vi "2015 Dumping.vi"(6 "Scoop angle":dbl format="%#_13g", 7 "Drum angle":dbl format="%#_13g", 8 "Winch angle":dbl, 9 "Dump":bool) -> (0 "Dumping Completed":bool, 1 "Drum PW":dbl format="%#_13g", 2 "Winch PW":dbl format="%#_13g", 3 "Scoop PW":dbl format="%#_13g")   [LabVIEW 2014]
panel:
  out "Numeric 2":i32
  out "Numeric":i32
  out "Boolean":bool
  out "Dump behav":bool
  out "D, S, W Aligned":bool
  # "Test indicators"
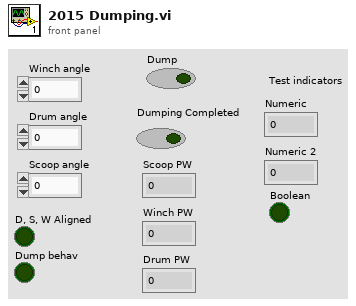
[diagram p1: front panel]
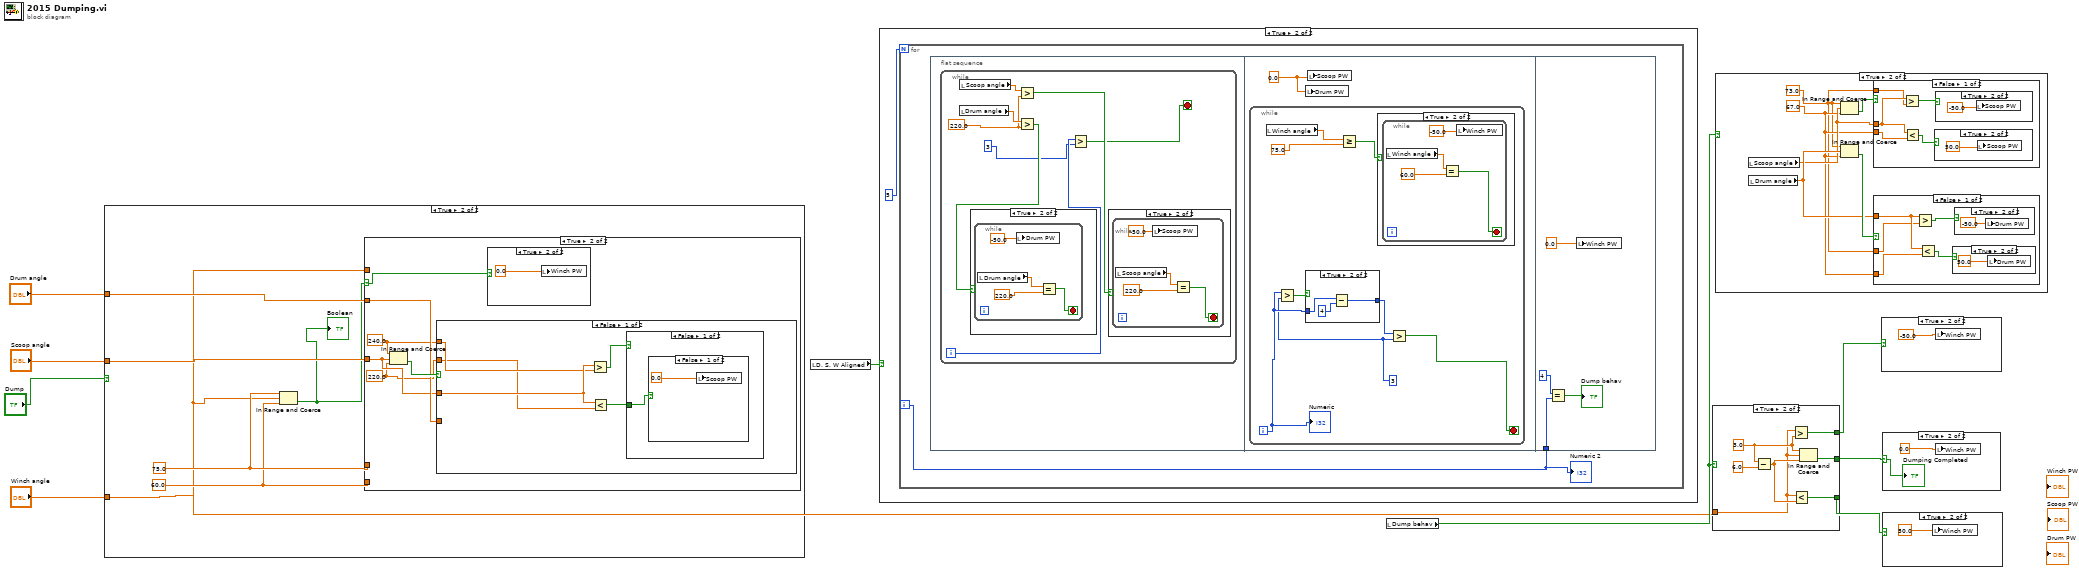
[diagram p0: block diagram]
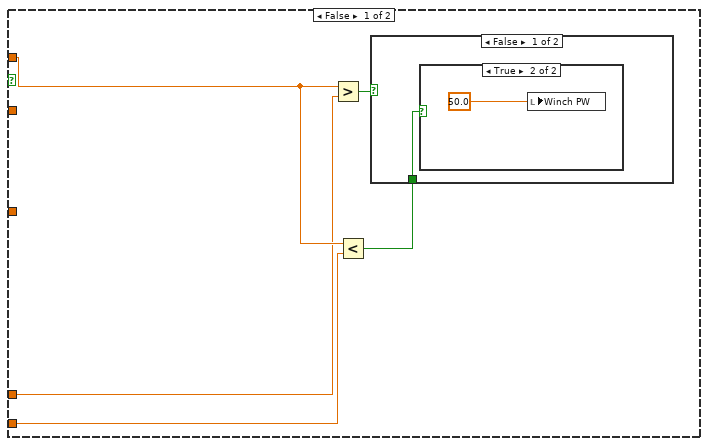
[diagram p3: hidden frame]
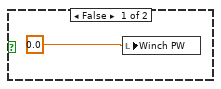
[diagram p4: hidden frame]
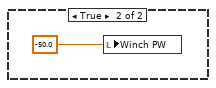
[diagram p5: hidden frame]
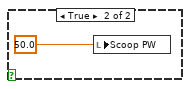
[diagram p7: hidden frame]
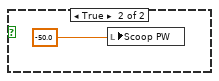
[diagram p8: hidden frame]
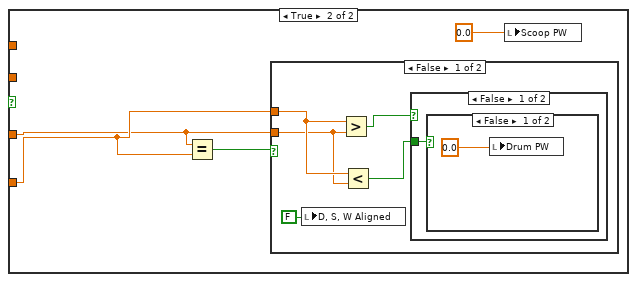
[diagram p9: hidden frame]
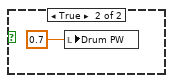
[diagram p10: hidden frame]
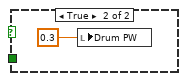
[diagram p11: hidden frame]
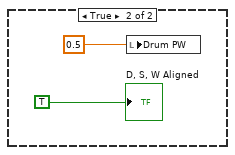
[diagram p12: hidden frame]
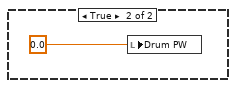
[diagram p16: hidden frame]
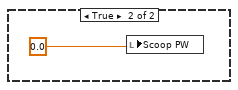
[diagram p19: hidden frame]
diagram:
  n1 = case shown="True" "Dump" {
    tunnel: "Drum angle" -> [_ w15]
    tunnel: "Scoop angle" -> [_ w14]
    tunnel: "Winch angle" -> [_ w11]
    frame False {
    }
    frame True {
      w12 = 60.0
      w13 = 75.0
      n2 = In Range and Coerce(upper limit=w13, x=w11, lower limit=w12) -> (In Range?=w10:bool)  [unwired: 1 out]
      "Boolean" <- w10
      n3 = case shown="True" w10 {
        selector: w10 -> [_ w27]
        tunnel: w15 -> [_ w29]
        tunnel: w11 -> [w19 _]
        tunnel: w13 -> [w18 _]
        tunnel: w12 -> [w17 _]
        tunnel: w14 -> [_ w28]
        frame False {
          n4 = Greater?(x=w19, y=w18) -> (0:w20:bool)
          n5 = Less?(x=w19, y=w17) -> (x < y?=w16:bool)
          n6 = case shown="False" w20 {
            tunnel: w16 -> [w21 _]
            frame False {
              n7 = case shown="True" w21 {
                frame False {
                  n8 = local write "Winch PW"(0.0) -> ()
                }
                frame True {
                  n9 = local write "Winch PW"(50.0) -> ()
                }
              }
            }
            frame True {
              n10 = local write "Winch PW"(-50.0) -> ()
            }
          }
        }
        frame True {
          w25 = 220.0
          w26 = 240.0
          n11 = In Range and Coerce(upper limit=w26, x=w28, lower limit=w25) -> (In Range?=w30:bool)  [unwired: 1 out]
          n12 = case shown="False" w30 {
            tunnel: w29 -> [_ w43]
            tunnel: w28 -> [w35 w41]
            tunnel: w26 -> [w34 _]
            tunnel: w25 -> [w33 _]
            frame False {
              n13 = Greater?(x=w35, y=w34) -> (0:w36:bool)
              n14 = Less?(x=w35, y=w33) -> (x < y?=w32:bool)
              n15 = case shown="False" w36 {
                tunnel: w32 -> [w37 _]
                frame False {
                  n16 = case shown="False" w37 {
                    frame False {
                      n17 = local write "Scoop PW"(0.0) -> ()
                    }
                    frame True {
                      n18 = local write "Scoop PW"(50.0) -> ()
                    }
                  }
                }
                frame True {
                  n19 = local write "Scoop PW"(-50.0) -> ()
                }
              }
            }
            frame True {
              n20 = Equal?(x=w41, y=w43) -> (x = y?=w42:bool)
              n21 = case shown="False" w42 {
                tunnel: w43 -> [w48 _]
                tunnel: w41 -> [w46 _]
                frame False {
                  n22 = local write "D, S, W Aligned"(FALSE) -> ()
                  n23 = Greater?(x=w48, y=w46) -> (0:w49:bool)
                  n24 = Less?(x=w48, y=w46) -> (x < y?=w45:bool)
                  n25 = case shown="False" w49 {
                    tunnel: w45 -> [w50 _]
                    frame False {
                      n26 = case shown="False" w50 {
                        frame False {
                          n27 = local write "Drum PW"(0.0) -> ()
                        }
                        frame True {
                          n28 = local write "Drum PW"(0.7) -> ()
                        }
                      }
                    }
                    frame True {
                      n29 = local write "Drum PW"(0.3) -> ()
                    }
                  }
                }
                frame True {
                  n30 = local write "Drum PW"(0.5) -> ()
                  "D, S, W Aligned" <- TRUE ("Boolean")
                }
              }
              n31 = local write "Scoop PW"(0.0) -> ()
            }
          }
          n32 = case shown="True" w27 {
            frame False {
            }
            frame True {
              n33 = local write "Winch PW"(0.0) -> ()
            }
          }
        }
      }
    }
  }
  n34 = local read "D, S, W Aligned"() -> (w4:bool)
  n35 = case shown="True" w4 {
    frame False {
    }
    frame True {
      n36 = for {
        N: 5 -> [_]
        i -> [w57]
        n37 = flat-sequence {
          tunnel: w57 -> [w103]
          frame #0 {
            n38 = while {
              i -> [w59]
              stop <- w60 stop-if-true
              w63 = 220.0
              n39 = local read "Drum angle"() -> (w65:dbl)
              n40 = local read "Scoop angle"() -> (w64:dbl)
              n41 = Greater?(x=w64, y=w63) -> (0:w62:bool)
              n42 = Greater?(x=w65, y=w63) -> (0:w61:bool)
              n43 = case shown="True" w61 {
                frame False {
                  n44 = while {
                    stop <- w66 stop-if-true
                    n45 = local read "Drum angle"() -> (w68:dbl)
                    n46 = local write "Drum PW"(50.0) -> ()
                    n47 = Equal?(x=w68, y=240.0) -> (x = y?=w66:bool)
                  }
                }
                frame True {
                  n48 = while {
                    stop <- w70 stop-if-true
                    n49 = local read "Drum angle"() -> (w72:dbl)
                    n50 = local write "Drum PW"(-50.0) -> ()
                    n51 = Equal?(x=w72, y=220.0) -> (x = y?=w70:bool)
                  }
                }
              }
              n52 = Greater?(x=w59, y=3) -> (0:w60:bool)
              n53 = case shown="True" w62 {
                frame False {
                  n54 = while {
                    stop <- w74 stop-if-true
                    n55 = local read "Scoop angle"() -> (w76:dbl)
                    n56 = local write "Scoop PW"(50.0) -> ()
                    n57 = Equal?(x=w76, y=240.0) -> (x = y?=w74:bool)
                  }
                }
                frame True {
                  n58 = while {
                    stop <- w78 stop-if-true
                    n59 = local read "Scoop angle"() -> (w80:dbl)
                    n60 = local write "Scoop PW"(-50.0) -> ()
                    n61 = Equal?(x=w80, y=220.0) -> (x = y?=w78:bool)
                  }
                }
              }
            }
          }
          frame #1 {
            w82 = 0.0
            n62 = while {
              i -> [w85]
              stop <- w87 stop-if-true
              w84 = 3
              n63 = local read "Winch angle"() -> (w90:dbl)
              n64 = Greater?(x=w85, y=w84) -> (0:w86:bool)
              n65 = case shown="True" w86 {
                tunnel: w85 -> [w91 w94]
                tunnel: [w91 w92] -> w83
                frame False {
                }
                frame True {
                  n66 = Subtract(x=w94, y=4) -> (x-y=w92:i32)
                }
              }
              n67 = Greater Or Equal?(x=w90, y=75.0) -> (x >= y?=w88:bool)
              n68 = case shown="True" w88 {
                frame False {
                  n69 = while {
                    stop <- w96 stop-if-true
                    n70 = local read "Winch angle"() -> (w98:dbl)
                    n71 = local write "Winch PW"(50.0) -> ()
                    n72 = Equal?(x=w98, y=75.0) -> (x = y?=w96:bool)
                  }
                }
                frame True {
                  n73 = while {
                    stop <- w99 stop-if-true
                    n74 = local read "Winch angle"() -> (w101:dbl)
                    n75 = Equal?(x=w101, y=60.0) -> (x = y?=w99:bool)
                    n76 = local write "Winch PW"(-50.0) -> ()
                  }
                }
              }
              n77 = Greater?(x=w83, y=w84) -> (0:w87:bool)
              "Numeric" <- w85
            }
            n78 = local write "Drum PW"(w82) -> ()
            n79 = local write "Scoop PW"(w82) -> ()
          }
          frame #2 {
            n80 = Equal?(x=4, y=w103) -> (x = y?=→"Dump behav":bool)
            n81 = local write "Winch PW"(0.0) -> ()
          }
        }
        "Numeric 2" <- w57
      }
    }
  }
  n82 = local read "Dump behav"() -> (w3:bool)
  n83 = case shown="True" w3 {
    tunnel: [w107 w112] -> w9
    tunnel: [w107 w111] -> w8
    tunnel: [w107 w110] -> w7
    tunnel: "Winch angle" -> [_ w108]
    frame False {
      w107 = FALSE
    }
    frame True {
      w109 = 3.0
      n84 = Subtract(x=w109, y=6.0) -> (x-y=w114:dbl)
      n85 = Greater?(x=w108, y=w109) -> (0:w112:bool)
      n86 = Less?(x=w108, y=w114) -> (x < y?=w110:bool)
      n87 = In Range and Coerce(upper limit=w109, x=w108, lower limit=w114) -> (In Range?=w111:bool)  [unwired: 1 out]
    }
  }
  n88 = case shown="True" w3 {
    frame False {
    }
    frame True {
      w116 = 67.0
      w115 = 73.0
      n89 = local read "Scoop angle"() -> (w117:dbl)
      n90 = local read "Drum angle"() -> (w118:dbl)
      n91 = In Range and Coerce(upper limit=w115, x=w117, lower limit=w116) -> (In Range?=w120:bool)  [unwired: 1 out]
      n92 = In Range and Coerce(upper limit=w115, x=w118, lower limit=w116) -> (In Range?=w119:bool)  [unwired: 1 out]
      n93 = case shown="False" w120 {
        tunnel: w117 -> [w133 _]
        tunnel: w115 -> [w131 _]
        tunnel: w116 -> [w132 _]
        frame False {
          n94 = Greater?(x=w133, y=w131) -> (0:w130:bool)
          n95 = Less?(x=w133, y=w132) -> (x < y?=w129:bool)
          n96 = case shown="True" w129 {
            frame False {
            }
            frame True {
              n97 = local write "Scoop PW"(50.0) -> ()
            }
          }
          n98 = case shown="True" w130 {
            frame False {
            }
            frame True {
              n99 = local write "Scoop PW"(-50.0) -> ()
            }
          }
        }
        frame True {
          n100 = local write "Scoop PW"(0.0) -> ()
        }
      }
      n101 = case shown="False" w119 {
        tunnel: w118 -> [w125 _]
        tunnel: w116 -> [w124 _]
        tunnel: w115 -> [w123 _]
        frame False {
          n102 = Greater?(x=w125, y=w123) -> (0:w121:bool)
          n103 = Less?(x=w125, y=w124) -> (x < y?=w122:bool)
          n104 = case shown="True" w122 {
            frame False {
            }
            frame True {
              n105 = local write "Drum PW"(50.0) -> ()
            }
          }
          n106 = case shown="True" w121 {
            frame False {
            }
            frame True {
              n107 = local write "Drum PW"(-50.0) -> ()
            }
          }
        }
        frame True {
          n108 = local write "Drum PW"(0.0) -> ()
        }
      }
    }
  }
  n109 = case shown="True" w9 {
    frame False {
    }
    frame True {
      n110 = local write "Winch PW"(-50.0) -> ()
    }
  }
  n111 = case shown="True" w8 {
    selector: w8 -> [_ w139]
    frame False {
    }
    frame True {
      n112 = local write "Winch PW"(0.0) -> ()
      "Dumping Completed" <- w139
    }
  }
  n113 = case shown="True" w7 {
    frame False {
    }
    frame True {
      n114 = local write "Winch PW"(50.0) -> ()
    }
  }
